vi "remoteControl.vi"() -> ()   [LabVIEW 2019]
uses:
  <vilib>/ReMiSYS/ReMiSYS_myRIO-mini/SubVI/gamepadF710/F710.ctl
  <vilib>/ReMiSYS/ReMiSYS_myRIO-mini/SubVI/gamepadF710/stick.ctl
  <vilib>/ReMiSYS/ReMiSYS_myRIO-mini/SubVI/gamepadF710/gamepadF710.lvclass
  <vilib>/Platform/TimedLoop/XDataNode/timing_clust.ctl
  <vilib>/Platform/TimedLoop/XDataNode/nitl_modes.ctl
  <vilib>/Platform/TimedLoop/XDataNode/wakeup.ctl
  <vilib>/ReMiSYS/ReMiSYS_myRIO-mini/SubVI/SYS/servoPort.ctl
  <vilib>/myRIO/Common/Instrument Driver Framework/myRIO v1.0/UART/vis/myRIO v1.0 Close UART.vi
  <vilib>/myRIO/Common/Instrument Driver Framework/Utilities/vis/FPGA Ref Manager.vi
  <vilib>/myRIO/Common/Instrument Driver Framework/myRIO v1.0/myRIO v1.0 Reset FPGA.vi
  <vilib>/myRIO/Common/Instrument Driver Framework/myRIO v1.0/IRQ/vis/myRIO v1.0 IRQ Info FGV.vi
  <vilib>/myRIO/Common/Instrument Driver Framework/myRIO v1.0/IRQ/vis/myRIO v1.0 Timer IRQ Info FGV.vi
  <vilib>/myRIO/Common/Instrument Driver Framework/myRIO v1.0/IRQ/vis/myRIO v1.0 ISR Agent.vi
  <vilib>/myRIO/Instrument Drivers/Utilities/vis/Reset Index.vi
  <vilib>/myRIO/Common/Instrument Driver Framework/myRIO v1.0/Resource Manager/vis/myRIO v1.0 Block Write Resource Manager.vi
  <vilib>/Platform/TimedLoop/XDataNode/XDataNode.xnode
  <vilib>/Platform/TimedLoop/XDataNode/XDNodeRunTimeDep.lvlib
  <vilib>/myRIO/Instrument Drivers/Utilities/Utilities.lvlib
panel:
  out "Image Out fgv 2":T1(plugin-control)
  out "Numeric Control":i32
  out "Position.y":sgl
  out "Position.x":sgl
  out "Image Out fgv":T1(plugin-control)
  out "shooterPitch":dbl
  out "ClipCtrl":bool[](array[boolean])
  out "Speed Array":dbl[](array[numeric])
  in  "stop Control?":bool
  out "F710":T2
  out "ENC [L, R, B] (deg)":dbl[](array[numeric])
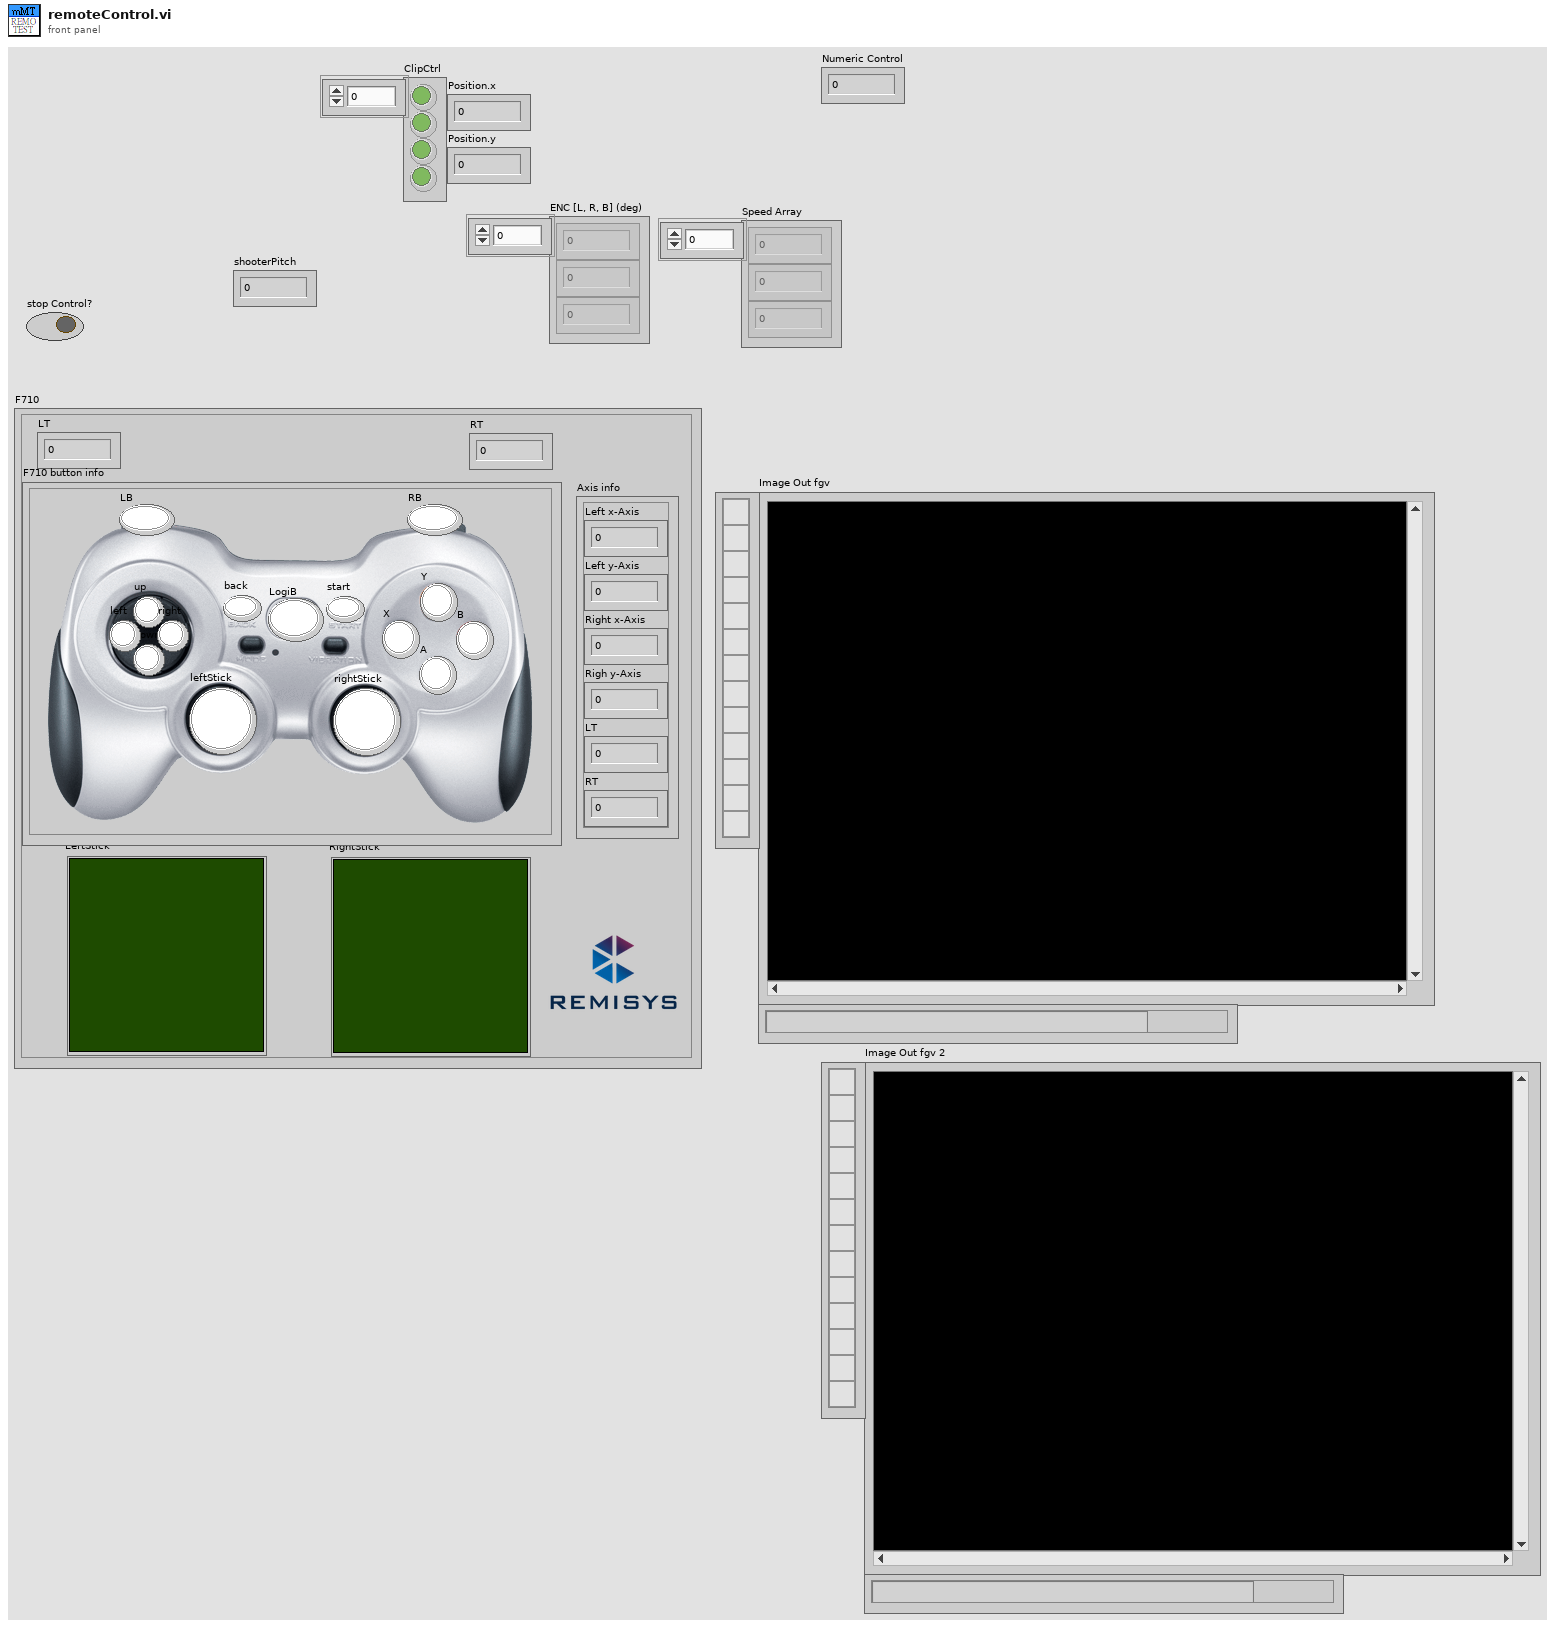
[diagram p1: front panel]
types:
  T1 = typedef "IMAQ Image.ctl" = refnum<image>
  T2 = typedef "F710.ctl" = cluster{"RT":u8, "LT":u8, "RightStick":T3, "LeftStick":T3, "Axis info":cluster{"Left x-Axis":i8, "Left y-Axis":i8, "Right x-Axis":i8, "Righ y-Axis":i8, "LT":u8, "RT":u8}, "F710 button info":cluster{"RB":bool, "LB":bool, "rightStick":bool, "leftStick":bool, "start":bool, "back":bool, "right":bool, "left":bool, "down":bool, "up":bool, "Y":bool, "X":bool, "B":bool, "A":bool, "LogiB":bool}}
  T3 = typedef "stick.ctl" = cluster{"X":dbl, "Y":dbl}[]
  T4 = cluster{"Position":cluster{"x":sgl, "y":sgl}, "Angle":sgl, "Scale":sgl, "Score":sgl, "Bounding Box":cluster{"x":sgl, "y":sgl}[]}
  T5 = typedef "IMAQ GM Match Report.ctl" = cluster{"Position":cluster{"x":sgl, "y":sgl}, "Angle":sgl, "Scale":sgl, "Score":sgl, "Bounding Box":cluster{"x":sgl, "y":sgl}[], "Contrast Reversed":bool, "Occlusion %":sgl, "Template Target Curve Score":sgl, "Target Template Curve Score":sgl, "Correlation Score":sgl}
  T6 = cluster{"Position":cluster{"x":sgl, "y":sgl}, "Angle":sgl, "Scale":sgl, "Score":sgl, "Bounding Box":cluster{"x":sgl, "y":sgl}[]}[]
  T7 = typedef "servoPort.ctl" = enum16{"S1", "S2", "S3", "S4", "S5", "S6", "S7", "S8", "S9"}
  T8 = typedef "XDNodeRunTimeDep.lvlib/timing_clust.ctl" = cluster{"Expected End [f-1]":u64, "Actual End [f-1]":u64, "Finished Late? [f-1]":bool, "Expected End [i-1]":u64, "Actual End [i-1]":u64, "Finished Late? [i-1]":bool, "Expected Start [i]":u64, "Actual Start [i]":u64, "Expected Start [f]":u64, "Actual Start [f]":u64, "Source Name":string, "Structure Name":string, "Period":i64, "Deadline":i64, "Offset":i64, "Start":i64, "Priority":i32, "Timeout":i32, "Mode":T9, "Wakeup Reason":T10, "Error":errorcluster, "Source Type":string, "Secondary Source Type":string, "Global End Time":u64, "Global Start Time":u64, "Frame Duration":u64, "Iteration Duration":u64, "Assigned CPU":i32, "I/O Scan Engine Mode":u32}
  T9 = typedef "XDNodeRunTimeDep.lvlib/nitl_modes.ctl" = enum32{"No Change", "Process missed periods, maintain original phase", "Discard missed periods, maintain original phase", "Process missed periods, ignore original phase", "Discard missed periods, ignore original phase"}
  T10 = typedef "XDNodeRunTimeDep.lvlib/wakeup.ctl" = enum32{"Normal", "Aborted", "Asynchronous wakeup", "Timing source error", "Timed loop error", "Timeout"}
  T11 = typedef "miniRef.ctl" = cluster{"Custom FPGA Reference":refnum<k20>, "error out":errorcluster}
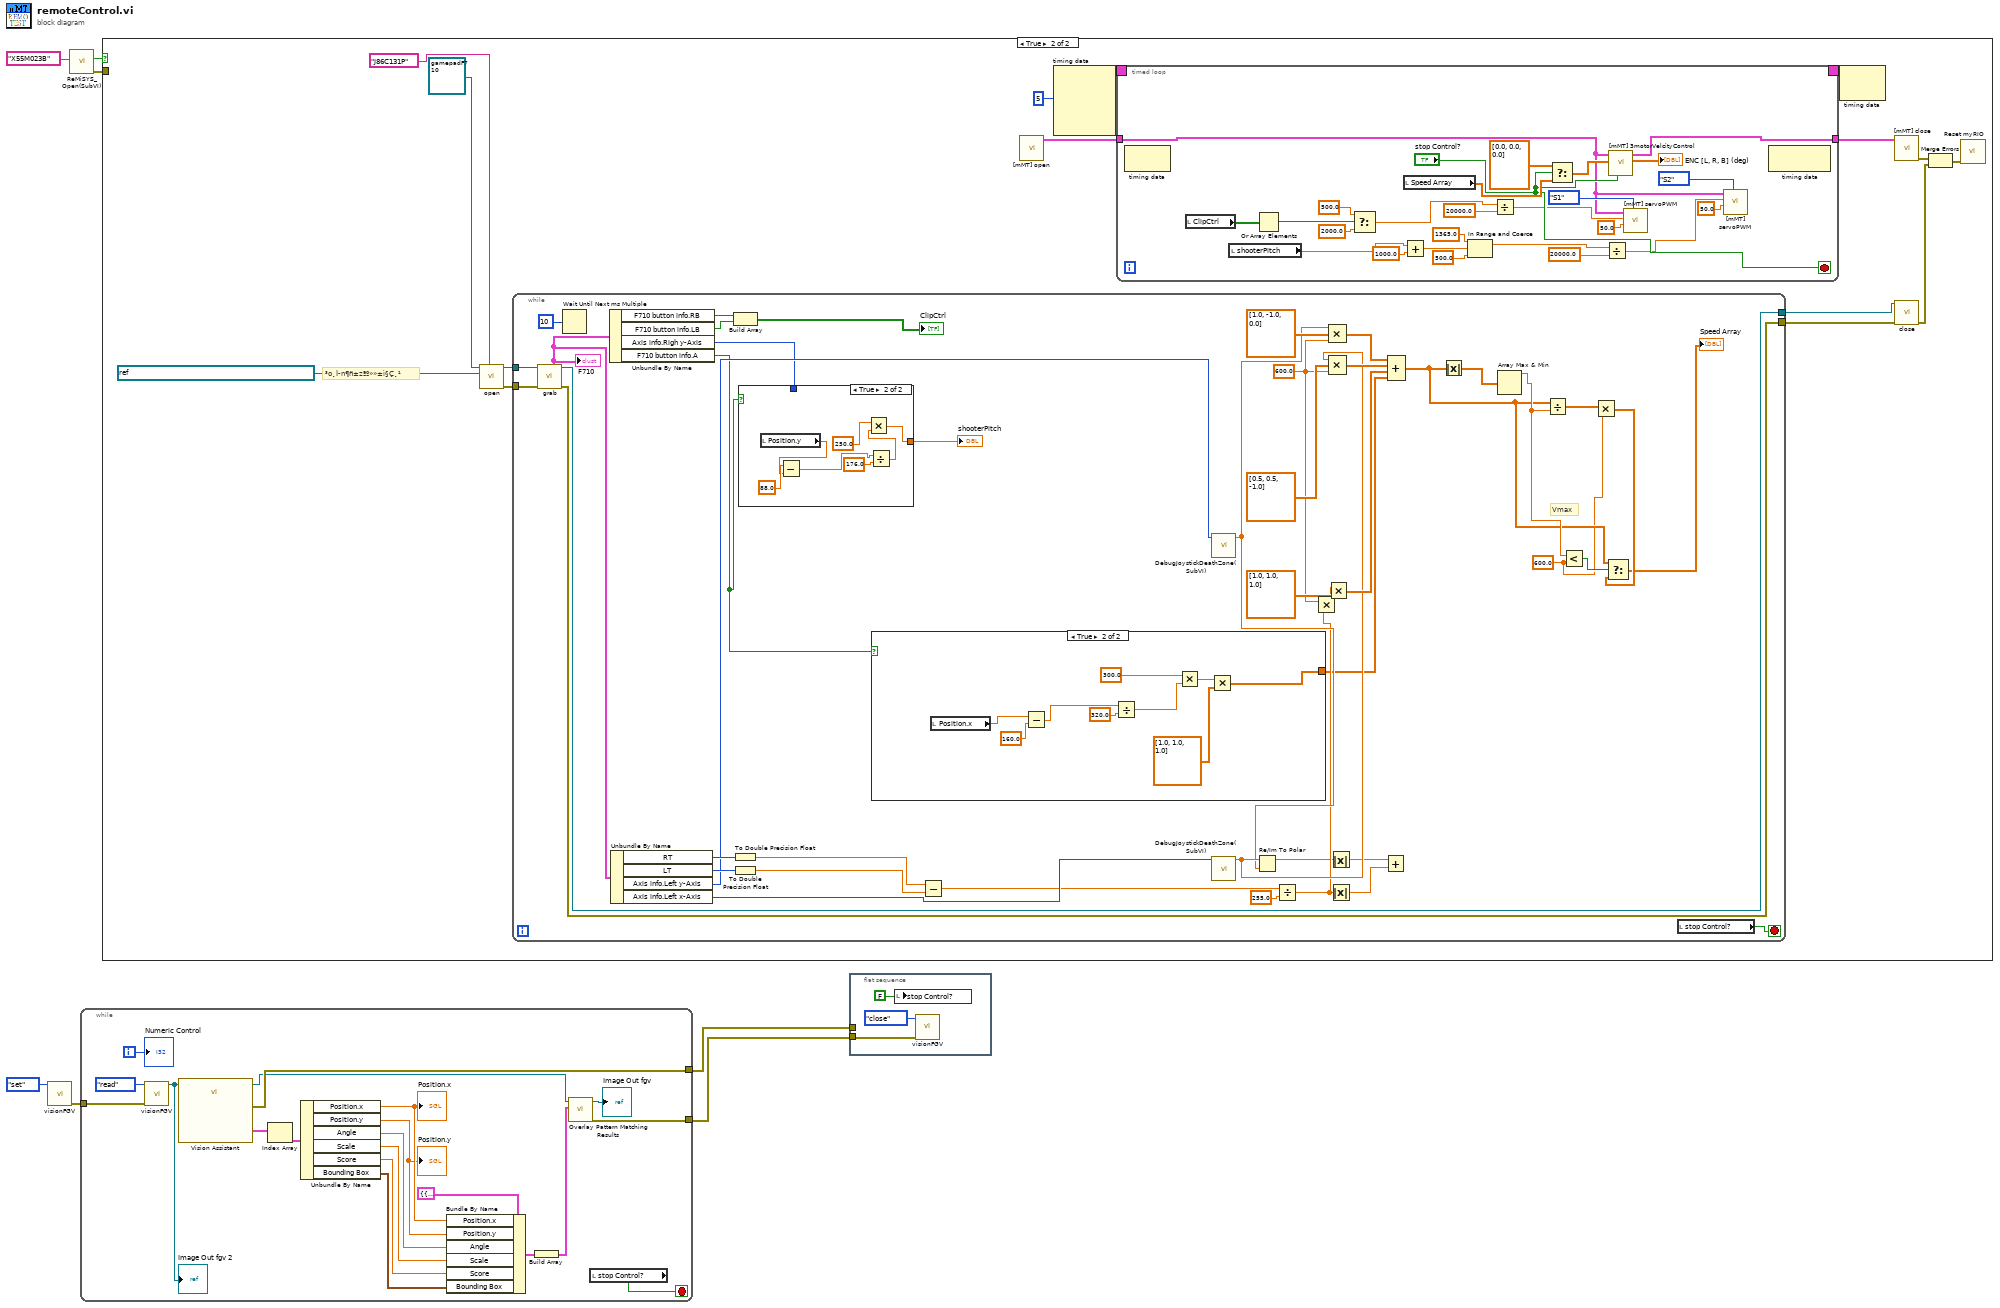
[diagram p0: block diagram]
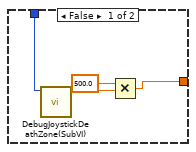
[diagram p3: hidden frame]
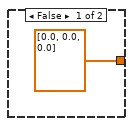
[diagram p4: hidden frame]
diagram:
  n1 = call "visionFGV.vi"("Function"=enum16{"set", "read", "close"}."set") -> ("error out"=w3:errorcluster)  [unwired: 9 in, 1 out]
  n2 = call <vilib>:"ReMiSYS_Open(SubVI).vi"("ReMiSYS Key"="X55M023B") -> ("error out"=w7:errorcluster, "Correct Key?"=w6:bool)  [unwired: 9 in]
  n3 = while {
    tunnel: w3 -> [w26]
    tunnel: [w24] -> w2
    tunnel: [w13] -> w1
    i -> [w9]
    stop <- w25 stop-if-true
    n4 = call "visionFGV.vi"("Error In"=w26, "Function"=enum16{"set", "read", "close"}."read") -> ("Image Out fgv"=w8:T1)  [unwired: 8 in, 1 out]
    "Image Out fgv 2" <- w8
    n5 = call "Vision Assistant"("Image In"=w8) -> ("Image Out"=w23:T1, "Matches (Pattern Matching 1)"=w22:T5[], "error out"=w24:errorcluster)  [unwired: 24 in]
    n6 = Index Array(array=w22) -> (element=w21:T5)  [unwired: 1 in]
    n7 = Unbundle By Name(w21) -> ("Position.x"=w20:sgl, "Position.y"=w19:sgl, "Angle"=w18:sgl, "Scale"=w17:sgl, "Score"=w16:sgl, "Bounding Box"=w15:cluster{"x":sgl, "y":sgl}[])
    "Position.x" <- w20
    "Position.y" <- w19
    n8 = Bundle By Name(cluster=T4 {"Position"={"x"=0.0, "y"=0.0}, "Angle"=0.0, "Scale"=0.0, "Score"=0.0, "Bounding Box"=[]} ("element"), "Position.x"=w20, "Position.y"=w19, "Angle"=w18, "Scale"=w17, "Score"=w16, "Bounding Box"=w15) -> (w14:T4)
    n9 = Build Array(w14) -> (w10:T6)
    n10 = call "Overlay Pattern Matching Results.vi"("Matches"=w10, "Image"=w23) -> ("error out"=w13:errorcluster, "Image Out"=→"Image Out fgv":T1)  [unwired: 8 in]
    n11 = local read "stop Control?"() -> (w25:bool)
    "Numeric Control" <- w9
  }
  n12 = case shown="True" w6 {
    tunnel: w7 -> [_ _]
    frame False {
    }
    frame True {
      # "³o¸Ì­n¶ñ±zªº»»±ì§Ç¸¹"
      n13 = call <vilib>:"open.vi"("INPUT S/N"="J86C131P", "VISA resource name"=refnum<visa-resource-name> "USB0::0x046D::0xC21F::D85E9710::RAW", "gamepadF710 in"=refnum<class "gamepadF710.lvclass"> refnum) -> ("error out"=w33:errorcluster, "gamepadF710 out"=w37:refnum<class "gamepadF710.lvclass">)  [unwired: 7 in]
      n14 = while {
        tunnel: w37 -> [w86]
        tunnel: [w85] -> w36
        tunnel: w33 -> [w57]
        tunnel: [w56] -> w32
        stop <- w84 stop-if-true
        w50 = 600.0 ("y")
        w46 = 600.0 ("tiltScale")
        # "Vmax"
        n15 = call <vilib>:"grab.vi"("error in (no error)"=w57, "gamepadF710 in"=w86) -> ("error out"=w56:errorcluster, "gamepadF710 out"=w85:refnum<class "gamepadF710.lvclass">, "F710"=w72:T2)  [unwired: 6 in]
        "F710" <- w72
        n16 = Wait Until Next ms Multiple(millisecond multiple=u32 10) -> ()  [unwired: 1 out]
        n17 = Unbundle By Name(w72) -> ("F710 button info.RB"=w71:bool, "F710 button info.LB"=w70:bool, "Axis info.Righ y-Axis"=w45:i8, "F710 button info.A"=w43:bool)
        n18 = Unbundle By Name(w72) -> ("RT"=w76:u8, "LT"=w74:u8, "Axis info.Left y-Axis"=w68:i8, "Axis info.Left x-Axis"=w67:i8)
        n19 = Build Array(w71, w70) -> (→"ClipCtrl":bool[])
        n20 = To Double Precision Float(number=w76) -> (double precision float=w75:dbl)
        n21 = To Double Precision Float(number=w74) -> (double precision float=w73:dbl)
        n22 = case shown="True" w43 {
          tunnel: w45 -> [w90 _]
          tunnel: [w87 w91] -> w44
          frame False {
            n23 = call <vilib>:"DebugJoystickDeathZone(SubVI).vi"("Axis_Info"=w90) -> ("ValueOut 1~-1"=w89:dbl)  [unwired: 10 in]
            n24 = Multiply(x=500.0, y=w89) -> (x*y=w87:dbl)
          }
          frame True {
            n25 = local read "Position.y"() -> (w95:sgl)
            n26 = Subtract(x=sgl 88.0 ("y"), y=w95) -> (x-y=w94:sgl)
            n27 = Divide(x=w94, y=176.0) -> (x/y=w93:dbl)
            n28 = Multiply(x=250.0 ("pitchSpeed"), y=w93) -> (x*y=w91:dbl)
          }
        }
        "shooterPitch" <- w44
        n29 = case shown="True" w43 {
          tunnel: [dbl[] [0.0, 0.0, 0.0] w104] -> w55
          frame False {
          }
          frame True {
            n30 = local read "Position.x"() -> (w107:sgl)
            n31 = Subtract(x=w107, y=sgl 160.0) -> (x-y=w100:sgl)
            n32 = Divide(x=w100, y=320.0) -> (x/y=w99:dbl)
            n33 = Multiply(x=sgl 300.0 ("turnSpeed"), y=w99) -> (x*y=w103:dbl)
            n34 = Multiply(x=w103, y=dbl[] [1.0, 1.0, 1.0]) -> (x*y=w104:dbl[])
          }
        }
        n35 = Subtract(x=w75, y=w73) -> (x-y=w66:dbl)
        n36 = call <vilib>:"DebugJoystickDeathZone(SubVI).vi"("Axis_Info"=w68) -> ("ValueOut 1~-1"=w63:dbl)  [unwired: 10 in]
        n37 = call <vilib>:"DebugJoystickDeathZone(SubVI).vi"("Axis_Info"=w67) -> ("ValueOut 1~-1"=w64:dbl)  [unwired: 10 in]
        n38 = Re/Im To Polar(2:w63, 3:w64) -> (1:w61:dbl)  [unwired: 1 out]
        n39 = Divide(x=w66, y=255.0) -> (x/y=w62:dbl)
        n40 = Multiply(x=w46, y=w62) -> (x*y=w47:dbl)
        n41 = Multiply(x=w47, y=dbl[] [1.0, 1.0, 1.0]) -> (x*y=w77:dbl[])
        n42 = Compound Arithmetic op=MULTIPLY(w63, dbl[] [1.0, -1.0, 0.0], w46) -> (w79:dbl[])
        n43 = Compound Arithmetic op=MULTIPLY(w64, dbl[] [0.5, 0.5, -1.0], w46) -> (w78:dbl[])
        n44 = Absolute Value(x=w61) -> (abs(x)=w60:dbl)
        n45 = Absolute Value(x=w62) -> (abs(x)=w59:dbl)
        n46 = Add(x=w60, y=w59) -> ()  [unwired: 1 out]
        n47 = Compound Arithmetic op=ADD(w79, w78, w77, w55) -> (w52:dbl[])
        n48 = Absolute Value(x=w52) -> (abs(x)=w58:dbl[])
        n49 = Array Max & Min(array=w58) -> (max value=w53:dbl)  [unwired: 3 out]
        n50 = Divide(x=w52, y=w53) -> (x/y=w51:dbl[])
        n51 = Less?(x=w53, y=w50) -> (x < y?=w54:bool)
        n52 = Multiply(x=w51, y=w50) -> (x*y=w49:dbl[])
        n53 = Select(t=w52, s=w54, f=w49) -> (s? t:f=→"Speed Array":dbl[])
        n54 = local read "stop Control?"() -> (w84:bool)
      }
      n55 = call <vilib>:"[mMT] open.vi"() -> ("miniOut"=w40:T11)  [unwired: 9 in, 2 out]
      n56 = node-c288(i64 5 ("Period")) -> (w42:T8)  [unwired: 3 in]
      n57 = timed-loop {
        tunnel: w40 -> [w123]
        timing: w42 -> [_]
        timing-out: [_] -> w41
        tunnel: [w133] -> w39
        stop <- "stop Control?" stop-if-true
        n58 = node-c288() -> ()  [unwired: 1 in, 1 out]
        n59 = local read "ClipCtrl"() -> (w118:bool[])
        n60 = local read "shooterPitch"() -> (w108:dbl)
        n61 = Or Array Elements(Boolean array=w118) -> (logical OR=w117:bool)
        n62 = Select(t=500.0 ("y"), s=w117, f=2000.0 ("y")) -> (s? t:f=w110:dbl)
        n63 = local read "Speed Array"() -> (w131:dbl[])
        n64 = Add(x=w108, y=1000.0) -> (x+y=w119:dbl)
        n65 = In Range and Coerce(upper limit=1365.0, x=w119, lower limit=500.0) -> (coerced(x)=w113:dbl)  [unwired: 1 out]
        n66 = Divide(x=w110, y=20000.0) -> (x/y=w109:dbl)
        n67 = Select(t=dbl[] [0.0, 0.0, 0.0], s="stop Control?", f=w131) -> (s? t:f=w129:dbl[])
        n68 = Divide(x=w113, y=20000.0) -> (x/y=w114:dbl)
        n69 = call <vilib>:"[mMT] 3motorVelcityControl.vi"("reset?"="stop Control?", "Speed [L, R, B] (deg/s)"=w129, "miniOut in"=w123) -> ("ENC [L, R, B] (deg)"=→"ENC [L, R, B] (deg)":dbl[], "miniOut out"=w133:T11)  [unwired: 5 in, 2 out]
        n70 = call <vilib>:"[mMT] servoPWM.vi"("servoPort"=servoPort."S1", "Frequency"=50.0, "DutyCycle"=w109, "miniOut in"=w123) -> ()  [unwired: 6 in, 2 out]
        n71 = call <vilib>:"[mMT] servoPWM.vi"("servoPort"=servoPort."S2", "Frequency"=50.0, "DutyCycle"=w114, "miniOut in"=w123) -> ()  [unwired: 6 in, 2 out]
        n72 = node-c288() -> ()  [unwired: 1 in, 1 out]
      }
      n73 = node-c288(w41) -> ()  [unwired: 1 out]
      n74 = call <vilib>:"[mMT] close.vi"("miniOut in"=w39) -> ("error out"=w31:errorcluster)  [unwired: 10 in]
      n75 = call <vilib>:"close.vi"("error in (no error)"=w32, "gamepadF710 in"=w36) -> ("error out"=w30:errorcluster)  [unwired: 8 in, 1 out]
      n76 = Merge Errors(w31, w30) -> (w29:errorcluster)
      n77 = call <vilib>:"Reset myRIO.vi"("error in (no error)"=w29) -> ()  [unwired: 10 in, 1 out]
    }
  }
  n78 = flat-sequence {
    tunnel: w2 -> [_]
    tunnel: w1 -> [w140]
    frame #0 {
      n79 = local write "stop Control?"(FALSE ("Stop Button")) -> ()
      n80 = call "visionFGV.vi"("Error In"=w140, "Function"=enum16{"set", "read", "close"}."close") -> ()  [unwired: 8 in, 2 out]
    }
  }
